vi "save_and_process_continious_image_data.vi"(4 "Path":path=path "C:/Users/MPI/Desktop", 8 "Save":bool, 9 "Enable online recon":bool, 11 "queue in":refnum<queue>) -> ()   [LabVIEW 2019]
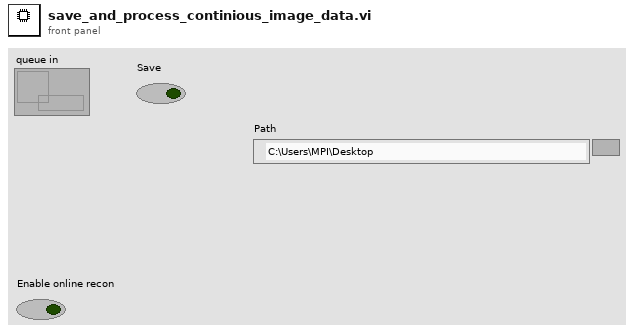
[diagram p1: front panel]
types:
  T1 = cluster{"Magnitude meas.":dbl[], "Phase meas.":dbl[], "Shift meas.":dbl[], "cw":bool, "projections per image":i32, "ramp-up readouts":i32, "current sense type":string, "Number of pulses per image":i32, "Rotation enabled":bool, "Rotary position":dbl[], "Baseline magnitude":dbl, "Baseline phase":dbl, "Wait readouts":i32, "Shift waveform type":string, "Shift enabled":bool, "Time domain data":dbl[], "Motor pulse duration":dbl, "Shift start":dbl, "Shift stop":dbl, "Notes":string, "Reconstructed image":picture, "Rotary encoder type":string, "Image start":timestamp, "Image stop":timestamp, "readouts per projection":i32, "Recon enabled":bool, "Bidirectional shift":bool, "Imager mode":string, "Shift delay":dbl, "Shift frequency":dbl, "Image time (calc)":dbl, "Initial encoder position":dbl, "Recon data":dbl[][], "Trigger line values":i32[], "Bed position":dbl, "Sample image":picture, "Patch amplitude":dbl, "Patch frequency":dbl, "Patch phase":dbl}
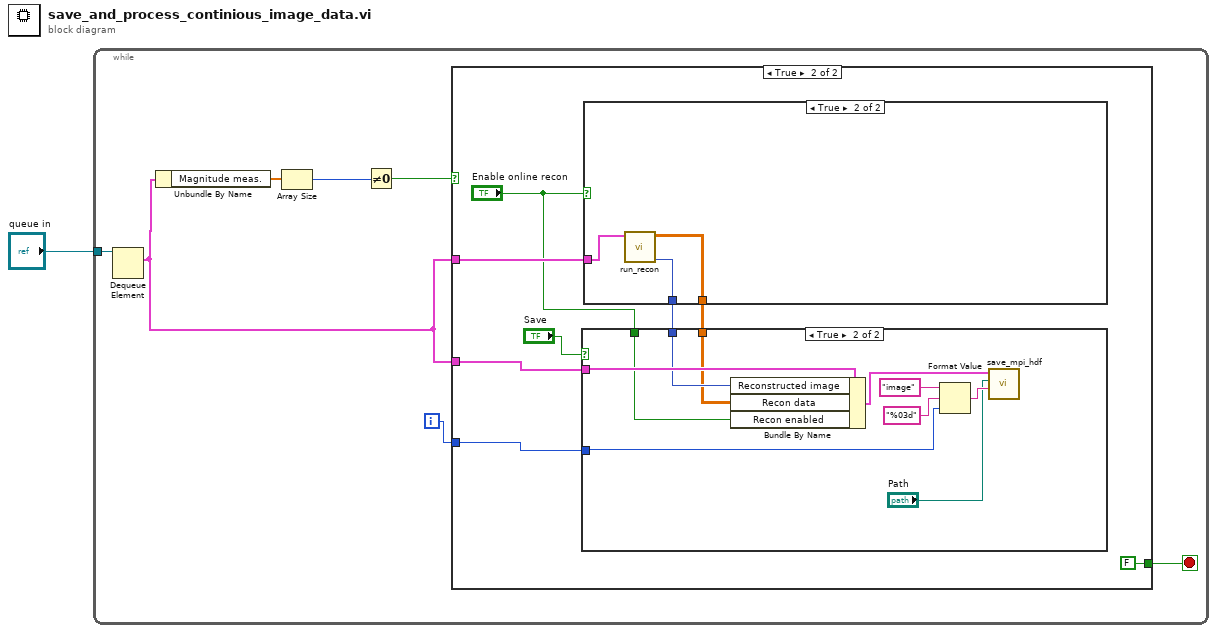
[diagram p0: block diagram]
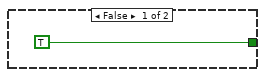
[diagram p2: hidden frame]
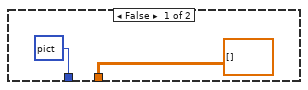
[diagram p3: hidden frame]
diagram:
  n1 = while {
    tunnel: "queue in" -> [w5]
    i -> [w3]
    stop <- w4 stop-if-true
    n2 = Dequeue Element(queue=w5) -> (element=w2:T1)  [unwired: 2 in, 3 out]
    n3 = Unbundle By Name(w2) -> ("Magnitude meas."=w8:dbl[])
    n4 = Array Size(array=w8) -> (size(s)=w7:i32)
    n5 = Not Equal To 0?(x=w7) -> (x != 0?=w6:bool)
    n6 = case shown="True" w6 {
      tunnel: [TRUE FALSE] -> w4
      tunnel: w3 -> [_ w16]
      tunnel: w2 -> [_ w15]
      tunnel: w2 -> [_ w14]
      frame False {
      }
      frame True {
        n7 = case shown="True" "Enable online recon" {
          tunnel: w15 -> [_ w20]
          tunnel: [picture data[5B] ("Reconstructed image") w22] -> w13
          tunnel: [dbl[][] [] ("Recon data") w21] -> w12
          frame False {
          }
          frame True {
            n8 = call "run_recon.vi"("Cluster in"=w20) -> ("reconstructed image"=w22:picture, "Recon data"=w21:dbl[][])  [unwired: 9 in]
          }
        }
        n9 = case shown="True" "Save" {
          tunnel: w16 -> [_ w30]
          tunnel: w14 -> [_ w28]
          tunnel: w13 -> [_ w26]
          tunnel: w12 -> [_ w25]
          tunnel: "Enable online recon" -> [_ w24]
          frame False {
          }
          frame True {
            n10 = Bundle By Name(cluster=w28, "Reconstructed image"=w26, "Recon data"=w25, "Recon enabled"=w24) -> (w27:T1)
            n11 = Format Value(string ("")="image", format string="%03d", value (0)=w30) -> (output string=w29:string)
            n12 = call "save_mpi_hdf.vi"("image dataset"=w29, "Path"="Path", "Cluster in"=w27) -> ()  [unwired: 9 in]
          }
        }
      }
    }
  }
